vi "mxwScript_Cmnd2Str_setDropRelation.vi"(8 "error in (no error)":errorcluster, 11 "data":variant) -> (0 "error out":errorcluster, 3 "outputString":string)   [LabVIEW 2020]
uses:
  codeGenAPISupport.llb/cgAPI_mxwScript_DrpTmplt_DropRelation.ctl
  codeGenAPISupport.llb/cgAPI_mxwScript_DrpTmplt_SimpleDirection.ctl
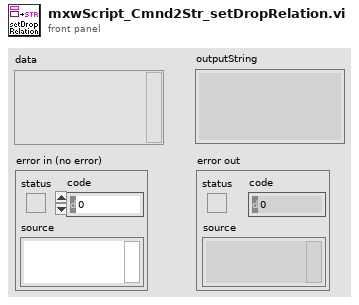
[diagram p1: front panel]
types:
  T1 = typedef "cgAPI_mxwScript_DrpTmplt_DropRelation.ctl" = cluster{"direction":T2, "distance":i32, "addWireSpace":bool}
  T2 = typedef "cgAPI_mxwScript_DrpTmplt_SimpleDirection.ctl" = enum16{"Right", "Left", "Below", "Above"}
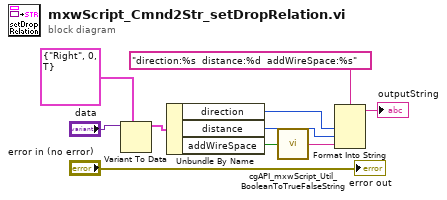
[diagram p0: block diagram]
diagram:
  n1 = Variant To Data(type=T1 {"direction"=enum."Right", "distance"=0, "addWireSpace"=TRUE} ("droptRelation"), Variant="data") -> (data=w8:T1)  [unwired: 1 in, 1 out]
  n2 = Unbundle By Name(w8) -> ("direction"=w4:T2, "distance"=w1:i32, "addWireSpace"=w3:bool)
  n3 = call "cgAPI_mxwScript_Util_BooleanToTrueFalseString.vi"("boolean"=w3) -> ("TRUE/FALSE text"=w2:string)  [unwired: 4 out]
  n4 = Format Into String(format string="direction:%s  distance:%d  addWireSpace:%s", w4, w1, w2) -> (resulting string=→"outputString":string)  [unwired: 2 in, 1 out]
  "error out" <- "error in (no error)"
